vi "Hydrosonic_Manual.vi"() -> ()   [LabVIEW 2012]
panel:
  in  "Mode":T1(ring)
  out "Tranducer Value":dbl format="%.2f"
  out "Transducer Error Info":string
  in  "Set Tranducer Value":T2(ring)
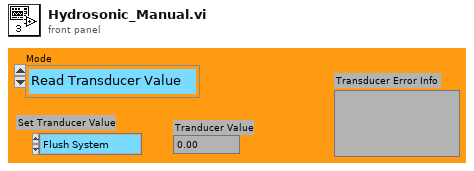
[diagram p1: front panel]
types:
  T1 = enum16{"Read Transducer Value", "Set Transducer value"}
  T2 = enum16{"Flush System", "0", "14", "29", "43", "57", "71", "86", "100"}
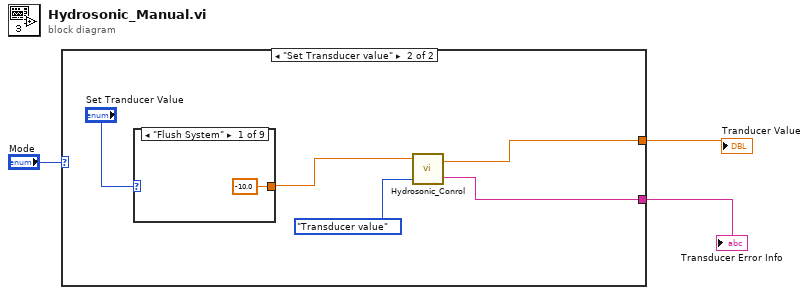
[diagram p0: block diagram]
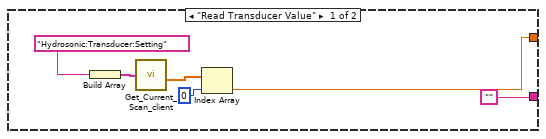
[diagram p2: hidden frame]
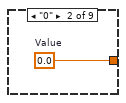
[diagram p3: hidden frame]
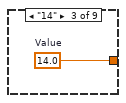
[diagram p4: hidden frame]
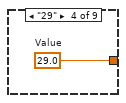
[diagram p5: hidden frame]
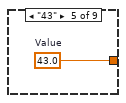
[diagram p6: hidden frame]
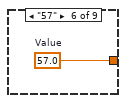
[diagram p7: hidden frame]
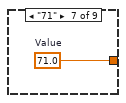
[diagram p8: hidden frame]
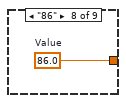
[diagram p9: hidden frame]
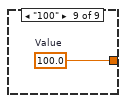
[diagram p10: hidden frame]
diagram:
  n1 = case shown="\"Set Transducer value\"" "Mode" {
    tunnel: [w4 w11] -> w3
    tunnel: ["" w10] -> w2
    frame "Read Transducer Value" {
      n2 = Build Array("Hydrosonic:Transducer:Setting") -> (w8:string[])
      n3 = call "Get_Current_Scan_client.vi"("ADAM Ch Names"=w8) -> ("Numerical Values"=w7:dbl[])  [unwired: 1 in, 2 out]
      n4 = Index Array(array=w7, index=0) -> (element=w4:dbl)
    }
    frame "Set Transducer value" {
      n5 = case shown="\"Flush System\"" "Set Tranducer Value" {
        tunnel: [-10.0 ("Value") w16 w17 w18 w19 w20 w21 w22 w23] -> w12
        frame "Flush System" {
        }
        frame "0" {
          w16 = 0.0  # Value
        }
        frame "14" {
          w17 = 14.0  # Value
        }
        frame "29" {
          w18 = 29.0  # Value
        }
        frame "43" {
          w19 = 43.0  # Value
        }
        frame "57" {
          w20 = 57.0  # Value
        }
        frame "71" {
          w21 = 71.0  # Value
        }
        frame "86" {
          w22 = 86.0  # Value
        }
        frame "100" {
          w23 = 100.0  # Value
        }
      }
      n6 = call "Hydrosonic_Conrol.vi"("Input Mode"=enum16{"Desired Frequency", "Transducer value"}."Transducer value", "Desired Value"=w12) -> ("Error Info"=w10:string, "Set output"=w11:dbl)  [unwired: 2 in]
    }
  }
  "Transducer Error Info" <- w2
  "Tranducer Value" <- w3
